vi "Write Data.vi"(8 "error in (no error)":errorcluster, 9 "Publication Time":timestamp, 10 "Value":variant, 11 "TerminalSignalingValueBinding In":refnum<class "TerminalSignalingValueBinding.lvclass">) -> (0 "error out":errorcluster, 3 "TerminalSignalingValueBinding Out":refnum<class "TerminalSignalingValueBinding.lvclass">)   [LabVIEW 2018, in "MVA Framework.lvlib" / "TerminalSignalingValueBinding.lvclass"]
doc: "写入数据"
uses:
  TerminalSignalingValueBinding.lvclass
  TerminalPropertyBinding/TerminalPropertyBinding.lvclass
  <vilib>/ErrorRing/Error Ring.xnode
  <vilib>/Utility/error.llb/Error Cluster From Error Code.vi
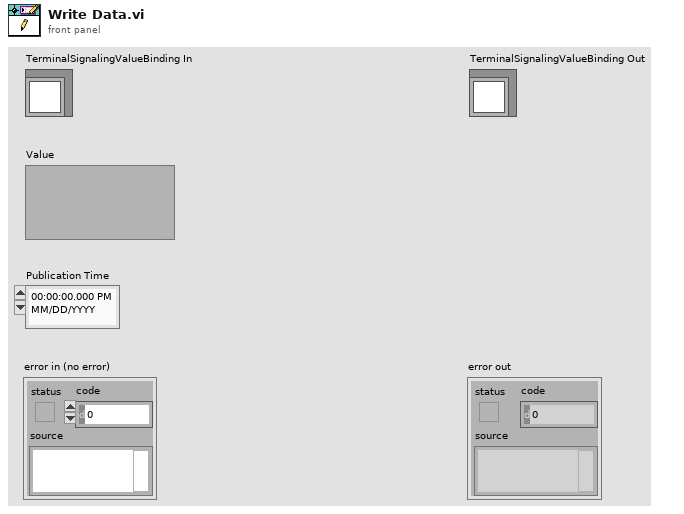
[diagram p1: front panel]
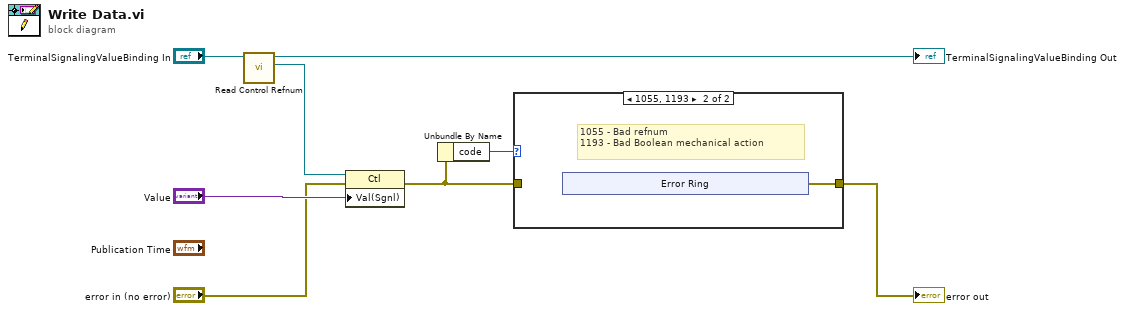
[diagram p0: block diagram]
diagram:
  n1 = call "Read Control Refnum.vi"("TerminalReferenceBinding in"="TerminalSignalingValueBinding In") -> ("Ctl Refnum"=w5:refnum<vi>, "TerminalReferenceBinding out"=→"TerminalSignalingValueBinding Out":refnum<class "TerminalSignalingValueBinding.lvclass">)  [unwired: 9 in]
  n2 = property class="Ctl"(reference=w5, error in="error in (no error)", "Val(Sgnl)"="Value") -> (error out=w2:errorcluster)  [unwired: 1 out]
  n3 = Unbundle By Name(w2) -> ("code"=w1:i32)
  n4 = case shown="1055, 1193" w1 {
    tunnel: w2 -> [w9 _]
    tunnel: [w9 w10] -> w3
    frame 0, Default {
    }
    frame 1055, 1193 {
      # "1055 - Bad refnum\n1193 - Bad Boolean mechanical action"
      n5 = xnode "Error Ring"() -> ("错误输出"=w10:errorcluster)
    }
  }
  "error out" <- w3
